vi "Read Instruments.vi"(8 "error in (no error)":errorcluster, 11 "Configuration in":refnum<class "Config.lvclass">) -> (0 "error out":errorcluster, 2 "Device List":string[](array[string]), 3 "Configuration out":refnum<class "Config.lvclass">)   [LabVIEW 2019]
doc: "Read device list from config.ini file"
uses:
  <vilib>/Utility/config.llb/NI_LVConfig.lvlib
  Config.lvclass
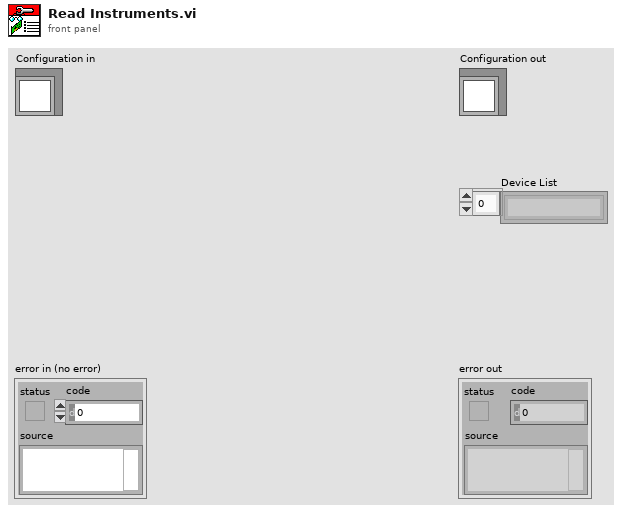
[diagram p1: front panel]
types:
  T1 = typedef "NI_LVConfig.lvlib/Config Data RefNum.ctl" = refnum<k1>
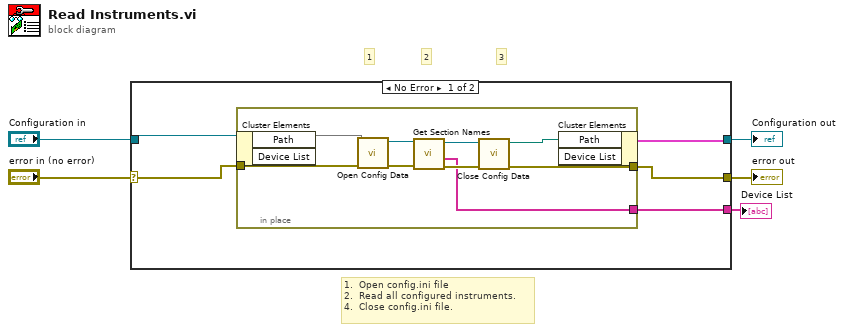
[diagram p0: block diagram]
diagram:
  # "1.  Open config.ini file\n2.  Read all configured instruments. \n4.  Close config.ini file."
  # "3"
  # "2"
  # "1"
  n1 = case shown="No Error" "error in (no error)" {
    selector: "error in (no error)" -> [w7 w21]
    tunnel: [w8 w21] -> w4
    tunnel: [w9 w20] -> w2
    tunnel: "Configuration in" -> [w10 w20]
    tunnel: [w6 _] -> w1
    frame No Error {
      n2 = in-place {
        in-place-border: [w13] -> w8
        in-place-border: w7 -> [w12]
        in-place-border: [w11] -> w6
        n3 = in-place-cluster #1(w10) -> ("Path"=w19)  [unwired: 1 out]
        n4 = call <vilib>:"Open Config Data.vi"("error in (no error)"=w12, "configuration file path"=w19) -> ("error out"=w18:errorcluster, "refnum"=w17:T1)  [unwired: 7 in, 1 out]
        n5 = call <vilib>:"Get Section Names.vi"("error in (no error)"=w18, "refnum"=w17) -> ("error out"=w14:errorcluster, "section names"=w11:string[], "refnum out"=w16:T1)  [unwired: 7 in]
        n6 = call <vilib>:"Close Config Data.vi"("error in (no error)"=w14, "refnum"=w16) -> ("error out"=w13:errorcluster, "file path"=w15:path)  [unwired: 8 in]
        n7 = in-place-cluster #1("Path"=w15) -> (w9:cluster{})  [unwired: 1 in]
      }
    }
    frame Error {
    }
  }
  "error out" <- w4
  "Configuration out" <- w2
  "Device List" <- w1
